vi "Export.vi"(8 "error in (no error)":errorcluster, 11 "Test Report in":refnum<class "Test Report.Default.lvclass">) -> (0 "error out":errorcluster, 3 "Test Report out":refnum<class "Test Report.Default.lvclass">)   [LabVIEW 2013, in "Caraya.lvlib" / "Test Report.Default.lvclass"]
uses:
  Test Report.Default.lvclass
  Test Report.Default.lvclass/Test Report.Default.ctl
  Test Report/Test Report.lvclass
  Test Result/Test Result.lvclass
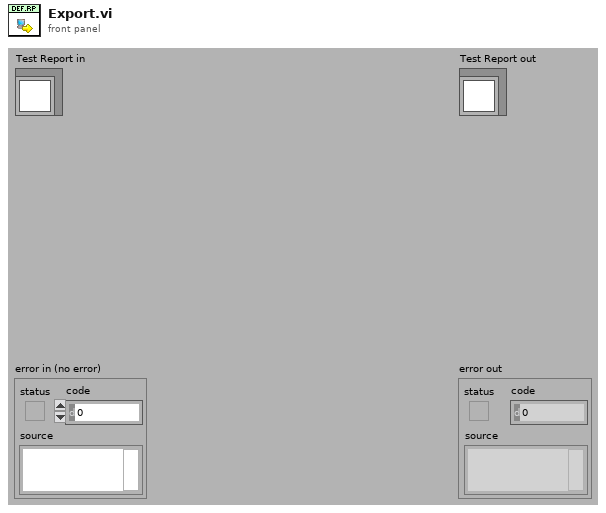
[diagram p1: front panel]
types:
  T1 = enum16{"open", "replace", "create", "open or create", "replace or create", "replace or create with confirmation"}
  T2 = typedef "Caraya.lvlib/Test Result.lvclass/Node Results.ctl" = cluster{"Node":T3, "Assertions":T5[]}
  T3 = typedef "Caraya.lvlib/Test Result.lvclass/Test Node.ctl" = cluster{"Test Registration":T4, "Defined":bool, "Passed":bool}
  T4 = typedef "Caraya.lvlib/Test Result.lvclass/Test Registration Data.ctl" = cluster{"Name":string, "Call Chain":string[], "Time Stamp":timestamp, "Test ID":string, "Caller ID":string}
  T5 = typedef "Caraya.lvlib/Test Result.lvclass/Assert Event Data.ctl" = cluster{"Name":string, "Passed":bool, "Call Chain":string[], "Test Error":errorcluster, "Time Stamp":timestamp, "Unique Assert ID":string, "Test ID":string, "Execution time (s)":dbl, "Verbose Explanation":string, "properties":variant, "measurements":variant, "limits":variant}
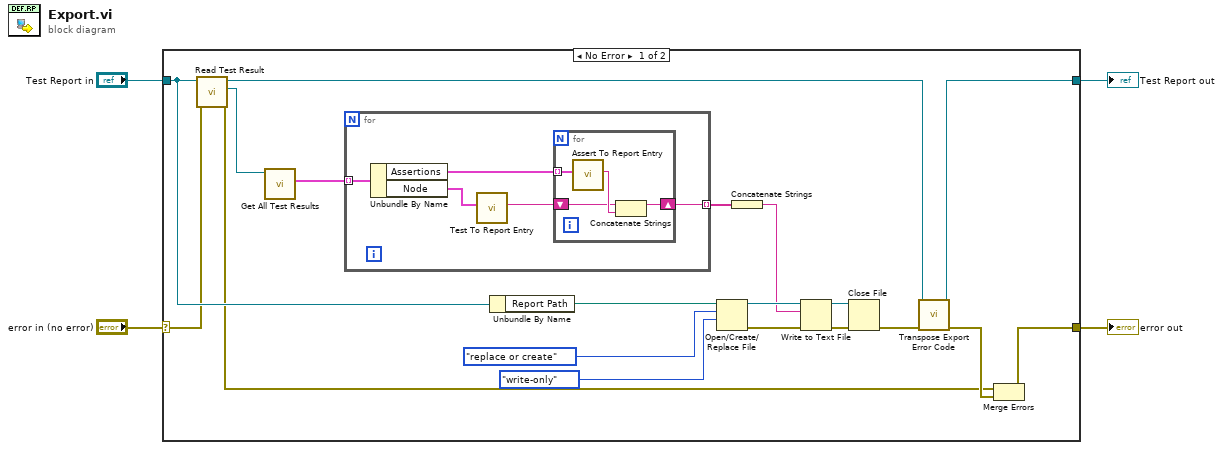
[diagram p0: block diagram]
diagram:
  n1 = case shown="No Error" "error in (no error)" {
    selector: "error in (no error)" -> [w15 w34]
    tunnel: [w9 w34] -> w3
    tunnel: [w5 w33] -> w1
    tunnel: "Test Report in" -> [w16 w33]
    frame No Error {
      n2 = call "Read Test Result.vi"("error in (no error)"=w15, "Test Report in"=w16) -> ("error out"=w8:errorcluster, "Caraya.lvlib:Test Result.lvclass"=w14:refnum<class "Test Result.lvclass">, "Test Report out"=w6:refnum<class "Test Report.Default.lvclass">)  [unwired: 7 in]
      n3 = call "Get All Test Results.vi"("Test Result in"=w14) -> ("Test Results"=w13:T2[])  [unwired: 8 in, 2 out]
      n4 = for {
        tunnel: w13 -> [w27] mode=indexing
        tunnel: [w25] -> w12 mode=indexing
        n5 = Unbundle By Name(w27) -> ("Assertions"=w24:T5[], "Node"=w26:T3)
        n6 = call "Test To Report Entry.vi"("Test Node"=w26) -> ("String"=w28:string)  [unwired: 9 in, 1 out]
        n7 = for {
          shift-right: [w29] -> w25
          shift-left: w28 -> [w30]
          tunnel: w24 -> [w32] mode=indexing
          n8 = call "Assert To Report Entry.vi"("Assert"=w32) -> ("String"=w31:string)  [unwired: 9 in, 1 out]
          n9 = Concatenate Strings(w30, w31) -> (w29:string)
        }
      }
      n10 = Unbundle By Name(w16) -> ("Report Path"=w17:path)
      n11 = Open/Create/Replace File(file path (use dialog)=w17, operation (0:open)=T1."replace or create", access (0:read/write)=enum16{"read/write", "read-only", "write-only"}."write-only") -> (refnum out=w21:refnum<file>, error out=w20:errorcluster)  [unwired: 3 in, 1 out]
      n12 = Concatenate Strings(w12) -> (w11:string)
      n13 = Write to Text File(file (use dialog)=w21, text=w11, error in=w20) -> (refnum out=w19:refnum<file>, error out=w18:errorcluster)  [unwired: 1 in, 1 out]
      n14 = Close File(refnum=w19, error in=w18) -> (error out=w7:errorcluster)  [unwired: 1 out]
      n15 = call-dynamic "Transpose Export Error Code.vi"("error in (no error)"=w7, "Test Report"=w6) -> ("error out"=w10:errorcluster, "Test Report out"=w5:refnum<class "Test Report.Default.lvclass">)  [unwired: 8 in]
      n16 = Merge Errors(w8, w10) -> (w9:errorcluster)
    }
    frame Error {
    }
  }
  "error out" <- w3
  "Test Report out" <- w1
